vi "SkewMatrix.vi"   [LabVIEW 2014]
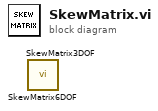
[diagram p0: block diagram]
diagram:
  n1 = call "SkewMatrix6DOF.vi"() -> ()  [unwired: 1 in, 1 out]
  n2 = call "SkewMatrix3DOF.vi"() -> ()  [unwired: 1 in, 1 out]
